vi "MAC qFREE.vi"(0 "System no.":i32=1 min=1 max=4 step=1, 5 "error in":errorcluster) -> (14 "No. of characters":i32, 19 "error out":errorcluster)   [LabVIEW 2026]
doc: "Returns the amount of free memory for macro recording (in number of characters).\n\nC-867: \n\nE-816: This command cannot be issued to a slave. Check controller manual to find out if MAC FREE? is supported.\n\nC-887, F-206, M-8X0: Only for GCS syntax version = GCS 2.0 or higher (check with CSV?.vi. If CSV?.vi is not supported, syntax version is GCS 1.0)."
panel:
  # "Returns the amount of free memory for macro recording \n(in number of characters)."
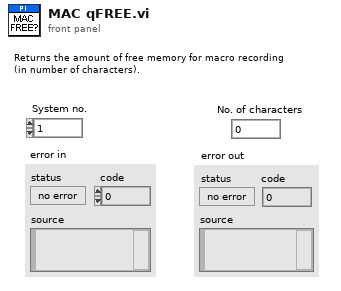
[diagram p1: front panel]
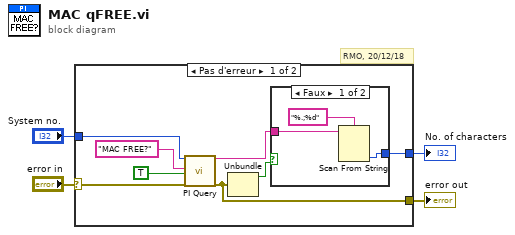
[diagram p0: block diagram]
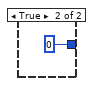
[diagram p2: hidden frame]
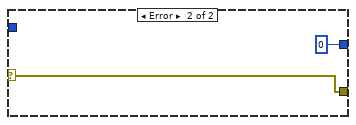
[diagram p3: hidden frame]
diagram:
  # "RMO, 20/12/18"
  n1 = case shown="Pas d'erreur" "error in" {
    selector: "error in" -> [w7 w18]
    tunnel: [w11 0] -> w4
    tunnel: [w6 w18] -> w3
    tunnel: "System no." -> [w9 _]
    frame No Error {
      n2 = call "PI Query.vi"("System no."=w9, "String to send"="MAC FREE?", "Attach termination char.?"=TRUE ("Attach Linefeed?"), "error in"=w7) -> ("String read"=w5:string, "error out"=w6:errorcluster)  [unwired: 3 in, 11 out]
      n3 = Unbundle(w6) -> ("status"=w12:bool)  [unwired: 2 out]
      n4 = case shown="Faux" w12 {
        tunnel: w5 -> [w15 _]
        tunnel: [w13 0] -> w11
        frame False {
          n5 = Scan From String(format string="%.;%d" ("Format String"), input string=w15) -> (output 1=w13:i32)  [unwired: 2 in, 4 out]
        }
        frame True {
        }
      }
    }
    frame Error {
    }
  }
  "error out" <- w3
  "No. of characters" <- w4
